vi "Conveyor Control Logic.vi"(11 "Run Feed System In":bool) -> (2 "Conveyor Motor Value Out":dbl, 3 "Run Feed System Out":bool)   [LabVIEW 2016]
uses:
  Global Variables/Refnum Names.vi
  Global Variables/Robot Status.vi
  Global Variables/Conveyor Calibrations.vi
panel:
  in  "Conveyor Motor Value":dbl
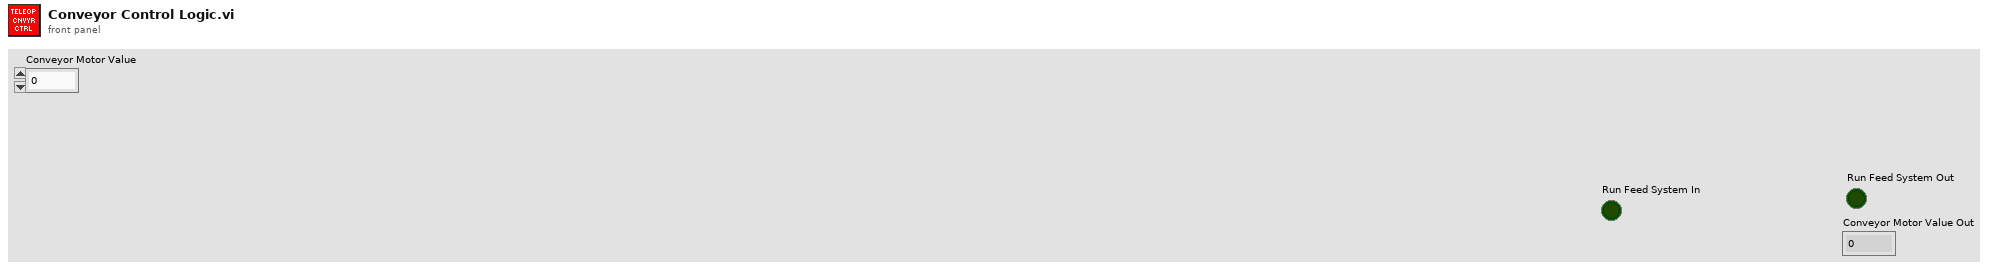
[diagram p1: front panel]
types:
  T1 = typedef "WPI_MotorControlDeviceRef.ctl" = cluster{"DeviceStatus":errorcluster, "Type":T2, "PWM":cluster{"PWM Channel":T3, "DeadBand":T4}, "CAN":cluster{"Device Number":u8, "SetOutput VI Ref":variant, "GetOutput VI Ref":variant, "Enable VI Ref":variant, "Disable VI Ref":variant, "Data":variant}, "Invert":bool}
  T2 = typedef "WPI_MotorControlType.ctl" = enum16{"PWM", "CAN"}
  T3 = typedef "FPGA_DIOPWMChannel.ctl" = enum8{"PWM 0", "PWM 1", "PWM 2", "PWM 3", "PWM 4", "PWM 5", "PWM 6", "PWM 7", "PWM 8", "PWM 9", "PWM MXP 0", "PWM MXP 1", "PWM MXP 2", "PWM MXP 3", "PWM MXP 4", "PWM MXP 5", "PWM MXP 6", "PWM MXP 7", "PWM MXP 8", "PWM MXP 9", "Invalid"}
  T4 = typedef "WPI_PWMDeadband.ctl" = cluster{"Name":string, "maxPositivePwm":i32, "minPositivePwm":i32, "centerPwm":i32, "maxNegativePwm":i32, "minNegativePwm":i32, "angularRange":u16}
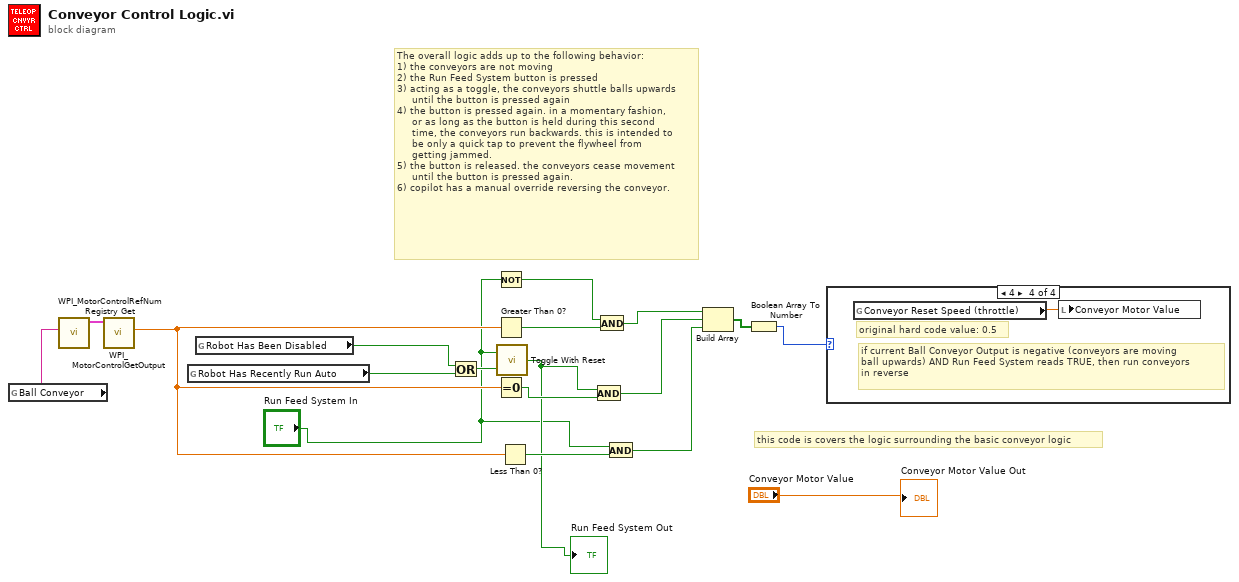
[diagram p0: block diagram]
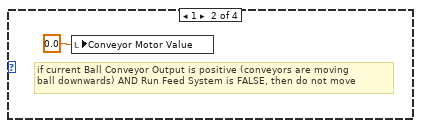
[diagram p3: hidden frame]
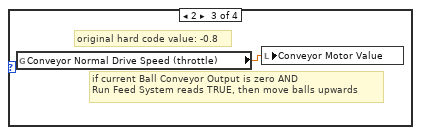
[diagram p4: hidden frame]
diagram:
  # "The overall logic adds up to the following behavior:\n1) the conveyors are not moving\n2) the Run Feed System button is pressed\n3) acting as a toggle, the conveyors shuttle balls upwards\n     until the button is pressed again\n4) the button is pressed again. in a momentary fashion,\n     or as long as the button is held during this second\n     time, the conveyors run backwards. this is intended to\n     be only a quick tap to prevent the flywheel from\n     getting jammed.\n5) the button is released. the conveyors cease movement\n     until the button is pressed again.\n6) copilot has a manual override reversing the conveyor."
  # "this code is covers the logic surrounding the basic conveyor logic"
  n1 = global read "Refnum Names.vi" "Ball Conveyor"() -> (w18:string)
  n2 = call <vilib>:"WPI_MotorControlRefNum Registry Get.vi"("refnum name"=w18) -> ("MotorControlDevRef"=w17:T1)  [unwired: 9 in, 1 out]
  n3 = call <vilib>:"WPI_MotorControlGetOutput.vi"("MotorControlDevRef"=w17) -> ("Output"=w16:dbl)  [unwired: 8 in, 2 out]
  n4 = global read "Robot Status.vi" "Robot Has Recently Run Auto"() -> (w11:bool)
  n5 = global read "Robot Status.vi" "Robot Has Been Disabled"() -> (w9:bool)
  n6 = Or(x=w9, y=w11) -> (x .or. y?=w10:bool)
  n7 = Not(x="Run Feed System In") -> (.not. x?=w14:bool)
  n8 = Greater Than 0?(x=w16) -> (x > 0?=w15:bool)
  n9 = Equal To 0?(x=w16) -> (x = 0?=w12:bool)
  n10 = call "Toggle With Reset.vi"("Reset"=w10, "Boolean"="Run Feed System In") -> ("Driver Switch 2"=w3:bool)
  "Run Feed System Out" <- w3
  n11 = Less Than 0?(x=w16) -> (x < 0?=w13:bool)
  n12 = And(x=w3, y=w12) -> (x .and. y?=w7:bool)
  n13 = And(x=w14, y=w15) -> (x .and. y?=w8:bool)
  n14 = And(x="Run Feed System In", y=w13) -> (x .and. y?=w6:bool)
  n15 = Build Array(w8, w7, w6) -> (w5:bool[])
  n16 = Boolean Array To Number(Boolean array=w5) -> (number=w4:u32)
  n17 = case shown="4" w4 {
    frame 0, Default {
    }
    frame 1 {
      # "if current Ball Conveyor Output is positive (conveyors are moving\nball downwards) AND Run Feed System is FALSE, then do not move"
      n18 = local write "Conveyor Motor Value"(0.0) -> ()
    }
    frame 2 {
      # "original hard code value: -0.8"
      # "if current Ball Conveyor Output is zero AND\nRun Feed System reads TRUE, then move balls upwards"
      n19 = global read "Conveyor Calibrations.vi" "Conveyor Normal Drive Speed (throttle)"() -> (w20:dbl)
      n20 = local write "Conveyor Motor Value"(w20) -> ()
    }
    frame 4 {
      # "if current Ball Conveyor Output is negative (conveyors are moving\nball upwards) AND Run Feed System reads TRUE, then run conveyors\nin reverse"
      # "original hard code value: 0.5"
      n21 = global read "Conveyor Calibrations.vi" "Conveyor Reset Speed (throttle)"() -> (w21:dbl)
      n22 = local write "Conveyor Motor Value"(w21) -> ()
    }
  }
  "Conveyor Motor Value Out" <- "Conveyor Motor Value"
